vi "Motion_Convert Home Data.vi"(10 "Home Data":T1 {"Position" format="%_7g"; "AccDec" format="%_7g"; "OffsetVelocity" format="%_7g"; "Offset" format="%_7g"; "Creep Velocity" format="%_7g"; "Approach Velocity" format="%_7g"}) -> (2 "Home Data":u16[](array[numeric]))   [LabVIEW 2010]
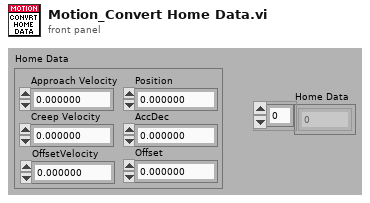
[diagram p1: front panel]
types:
  T1 = cluster{"Approach Velocity":dbl, "Creep Velocity":dbl, "Offset":dbl, "OffsetVelocity":dbl, "AccDec":dbl, "Position":dbl}
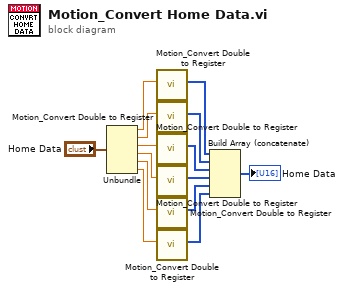
[diagram p0: block diagram]
diagram:
  n1 = Unbundle("Home Data") -> ("Approach Velocity"=w7:dbl, "Creep Velocity"=w6:dbl, "Offset"=w3:dbl, "OffsetVelocity"=w2:dbl, "AccDec"=w5:dbl, "Position"=w4:dbl)
  n2 = call "Motion_Convert Double to Register.vi"("Double Value"=w7) -> ("U16 Array"=w14:u16[])  [unwired: 10 in]
  n3 = call "Motion_Convert Double to Register.vi"("Double Value"=w6) -> ("U16 Array"=w13:u16[])  [unwired: 10 in]
  n4 = call "Motion_Convert Double to Register.vi"("Double Value"=w3) -> ("U16 Array"=w12:u16[])  [unwired: 10 in]
  n5 = call "Motion_Convert Double to Register.vi"("Double Value"=w2) -> ("U16 Array"=w11:u16[])  [unwired: 10 in]
  n6 = call "Motion_Convert Double to Register.vi"("Double Value"=w5) -> ("U16 Array"=w10:u16[])  [unwired: 10 in]
  n7 = call "Motion_Convert Double to Register.vi"("Double Value"=w4) -> ("U16 Array"=w9:u16[])  [unwired: 10 in]
  n8 = Build Array (concatenate)(w14, w13, w12, w11, w10, w9) -> (→"Home Data":u16[])
